vi "When Destroy.vi"(0 "error out":errorcluster, 11 "I2C Bus in":refnum<class "Mock I2C Bus.lvclass">) -> ()   [LabVIEW 2020, in "Mock I2C Bus.lvclass"]
uses:
  Mock I2C Bus.lvclass
  C:/Program Files (x86)/National Instruments/LabVIEW 2020/vi.lib/Astemes/LMock/Mock.lvclass
  <vilib>/Astemes/LMock/Mock.lvclass
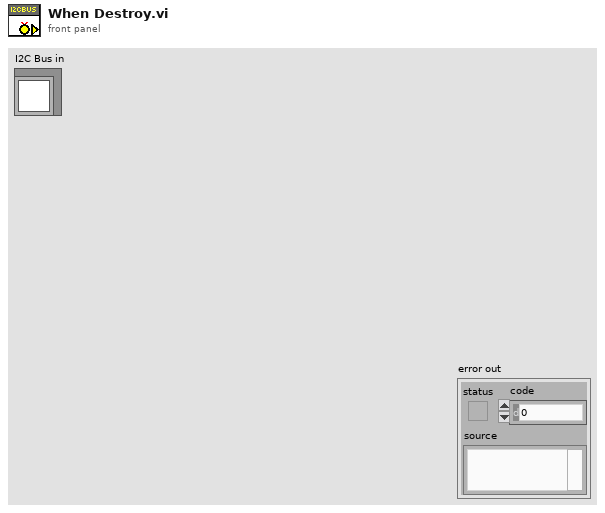
[diagram p1: front panel]
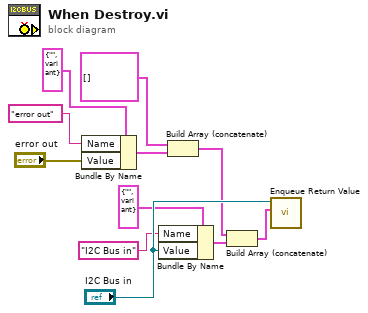
[diagram p0: block diagram]
diagram:
  n1 = Bundle By Name(cluster=cluster{"Name":string, "Value":variant} {"Name"="", "Value"=variant} ("element"), "Name"="error out", "Value"="error out") -> (w3:cluster{"Name":string, "Value":variant})
  n2 = Bundle By Name(cluster=cluster{"Name":string, "Value":variant} {"Name"="", "Value"=variant} ("element"), "Name"="I2C Bus in", "Value"="I2C Bus in") -> (w1:cluster{"Name":string, "Value":variant})
  n3 = Build Array (concatenate)(cluster{"Name":string, "Value":variant}[] [] ("Control Values"), w3) -> (w8:cluster{"Name":string, "Value":variant}[])
  n4 = Build Array (concatenate)(w8, w1) -> (w10:cluster{"Name":string, "Value":variant}[])
  n5 = call <vilib>:"Enqueue Return Value.vi"("Indicator Values"=w10, "Mock In"="I2C Bus in") -> ()  [unwired: 8 in, 2 out]
